vi "Test HDF5 chunk.vi"() -> ()   [LabVIEW 2012]
uses:
  <vilib>/addons/h5labview2/file/H5Fmode.ctl
  HDF5 append data (DBL 2D).vi
  <vilib>/addons/h5labview2/file/H5F.lvlib
  <vilib>/addons/h5labview2/group/H5G.lvlib
  <vilib>/addons/h5labview2/dataset/H5D.lvlib
panel:
  in  "file":path
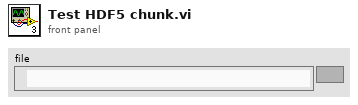
[diagram p1: front panel]
types:
  T1 = typedef "H5F.lvlib/H5Fmode.ctl" = enum16{"read-only", "read-write", "overwrite", "create new", "open or create"}
  T2 = typedef "hid_t.ctl" = i32
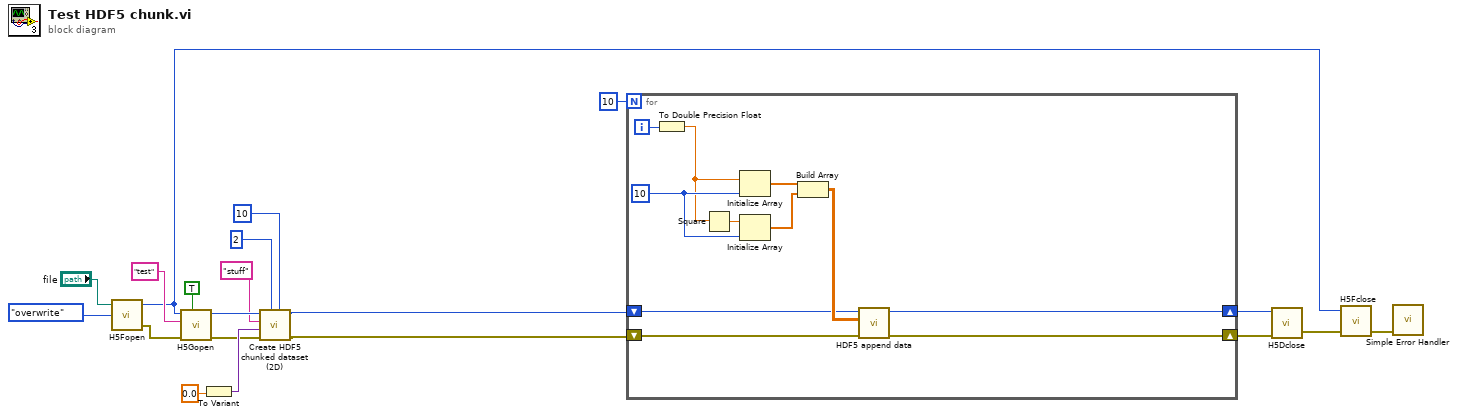
[diagram p0: block diagram]
diagram:
  n1 = call <vilib>:"H5Fopen.vi"("mode (read-only)"=H5Fmode."overwrite", "path"="file") -> ("error out"=w18:errorcluster, "ref out"=w12:T2)  [unwired: 2 in]
  n2 = call <vilib>:"H5Gopen.vi"("create? (F)"=TRUE, "error in (no error)"=w18, "name"="test", "ref in"=w12) -> ("error out"=w5:errorcluster, "group out"=w9:T2)  [unwired: 3 in]
  n3 = To Variant(anything=0.0) -> (Variant=w6:variant)
  n4 = call "Create HDF5 chunked dataset (2D).vi"("block size"=10, "number of channels"=2, "error in (no error)"=w5, "data type"=w6, "name"="stuff", "ref in"=w9) -> ("error out"=w1:errorcluster, "dset out"=w2:i32)  [unwired: 4 in]
  n5 = for {
    N: 10 -> [_]
    shift-right: [w30] -> w15
    shift-left: w2 -> [w21]
    shift-right: [w29] -> w14
    shift-left: w1 -> [w31]
    i -> [w26]
    w28 = u64 10 ("y")
    n6 = To Double Precision Float(number=w26) -> (double precision float=w25:dbl)
    n7 = Square(x=w25) -> (x^2=w27:dbl)
    n8 = Initialize Array(w25, w28) -> (w24:dbl[])
    n9 = Initialize Array(w27, w28) -> (w23:dbl[])
    n10 = Build Array(w24, w23) -> (w22:dbl[][])
    n11 = call-poly "HDF5 append data.vi"("error in (no error)"=w31, "data"=w22, "dset in"=w21) -> ("error out"=w29:errorcluster, "ref out"=w30:i32)  [unwired: 7 in]
  }
  n12 = call <vilib>:"H5Dclose.vi"("error in (no error)"=w14, "dset in"=w15) -> ("error out"=w13:errorcluster)  [unwired: 3 in]
  n13 = call <vilib>:"H5Fclose.vi"("error in (no error)"=w13, "ref"=w12) -> ("error out"=w10:errorcluster)  [unwired: 3 in]
  n14 = call <vilib>:"Simple Error Handler.vi"("error in (no error)"=w10) -> ()  [unwired: 4 in, 5 out]
